vi "lockin - Set REF phase equals zero.vi"(9 "reset REF phi to zero":bool, 10 "Channels: Lockin":T1={"REF f (Hz)"=[0.4, 0.4], "REF phi (°)"=[0.0, 0.0]} {"REF phi (°)" format="%#_3g"}, 11 "Channels: AO":T4={"AO amp (V)"=[0.0, 0.0, 0.0, 0.0, 0.0, 0.0, 0.0, 0.0], "AO DC (V)"=[0.0, 0.0, 0.0, 0.0, 0.0, 0.0, 0.0, 0.0], "AO f (Hz)"=[0.4, 0.4, 0.4, 0.4, 0.4, 0.4, 0.4, 0.4], "AO phi (°)"=[0.0, 0.0, 0.0, 0.0, 0.0, 0.0, 0.0, 0.0], "function"=[enum."Triangle", enum."Sine", enum."Sine", enum."Sine", enum."Sine", enum."Sine", enum."Sine", enum."Sine"], "I+"=[]} {"AO f (Hz)" min=0.001 max=10000.0; "AO DC (V)" format="%.3p"; "AO amp (V)" format="%.3p"}) -> (2 "Channels: Lockin 2":T1 {"REF phi (°)" format="%#_3g"}, 3 "Channels: AO 2":T4 {"AO f (Hz)" min=0.001 max=10000.0; "AO DC (V)" format="%.3p"; "AO amp (V)" format="%.3p"})   [LabVIEW 2016]
uses:
  Instrument.Lockin/Typedefs/REF-cluster.ctl
  Instrument.Lockin/Typedefs/REF_f-array.ctl
  Instrument.Lockin/Typedefs/REF_phi-array.ctl
  Instrument.Lockin/Typedefs/AO-cluster.ctl
  Instrument.Lockin/Typedefs/AO_Amp-array.ctl
  Instrument.Lockin/Typedefs/AO_DC-array.ctl
  Instrument.Lockin/Typedefs/AO_f-array.ctl
  Instrument.Lockin/Typedefs/AO_phi-array.ctl
  Instrument.Lockin/Typedefs/Function-array.ctl
  Instrument.Lockin/Typedefs/Function-enum.ctl
  Instrument.Lockin/Instrument.Lockin.lvclass
panel:
  # "1"
  # "2"
  # "3"
  # "4"
  # "5"
  # "6"
  # "7"
  # "8"
  # "1"
  # "2"
  # "3"
  # "4"
  # "5"
  # "6"
  # "7"
  # "8"
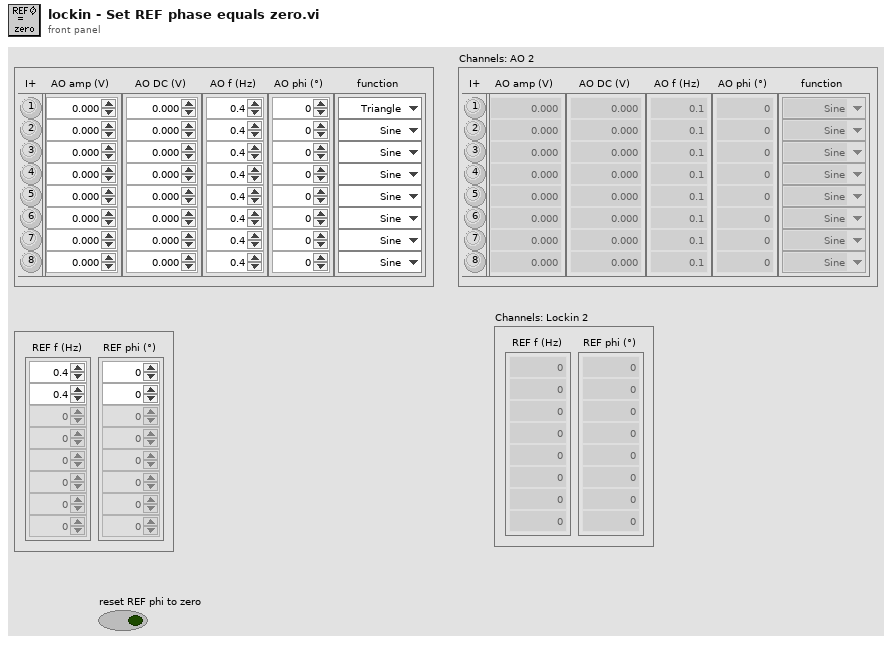
[diagram p1: front panel]
types:
  T1 = typedef "Instrument.Lockin.lvclass/REF-cluster.ctl" = cluster{"REF f (Hz)":T2, "REF phi (°)":T3}
  T2 = typedef "Instrument.Lockin.lvclass/REF_f-array.ctl" = dbl[]
  T3 = typedef "Instrument.Lockin.lvclass/REF_phi-array.ctl" = dbl[]
  T4 = typedef "Instrument.Lockin.lvclass/AO-cluster.ctl" = cluster{"AO amp (V)":T5, "AO DC (V)":T6, "AO f (Hz)":T7, "AO phi (°)":T8, "function":T9, "I+":bool[]}
  T5 = typedef "Instrument.Lockin.lvclass/AO_Amp-array.ctl" = dbl[]
  T6 = typedef "Instrument.Lockin.lvclass/AO_DC-array.ctl" = dbl[]
  T7 = typedef "Instrument.Lockin.lvclass/AO_f-array.ctl" = dbl[]
  T8 = typedef "Instrument.Lockin.lvclass/AO_phi-array.ctl" = dbl[]
  T9 = typedef "Instrument.Lockin.lvclass/Function-array.ctl" = T10[]
  T10 = typedef "Instrument.Lockin.lvclass/Function-enum.ctl" = enum16{"Sine", "Triangle", "Square", "Sawtooth"}
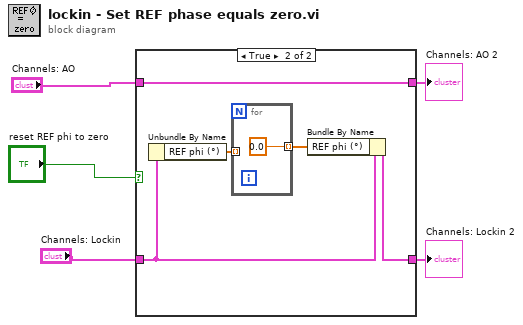
[diagram p0: block diagram]
diagram:
  n1 = case shown="True" "reset REF phi to zero" {
    tunnel: "Channels: AO" -> [w7 w10]
    tunnel: [w7 w10] -> w5
    tunnel: "Channels: Lockin" -> [w6 w9]
    tunnel: [w6 w8] -> w4
    frame False {
    }
    frame True {
      n2 = Unbundle By Name(w9) -> ("REF phi (°)"=w12:T3)
      n3 = for {
        tunnel: w12 -> [_] mode=indexing
        tunnel: [0.0] -> w11 mode=indexing
      }
      n4 = Bundle By Name(cluster=w9, "REF phi (°)"=w11) -> (w8:T1)
    }
  }
  "Channels: AO 2" <- w5
  "Channels: Lockin 2" <- w4
